vi "串口INI.vi"() -> ()   [LabVIEW 2019]
uses:
  <vilib>/Instr/_visa.llb/VISA Configure Serial Port (Instr).vi
panel:
  in  "启用终止符？":bool caption="启用终止符 (F)"
  in  "终止符":u8=10 format="%.0x"
  in  "超时":u32=10000 caption="超时（10秒）"
  in  "流控制":u16(ring) items=["无", "XON/XOFF", "RTS/CTS", "XON/XOFF & RTS/CTS", "DTR/DSR", "XON/XOFF & DTR/DSR"]
  in  "停止位":u16(ring)=10 items=["1.0"=10, "1.5"=15, "2.0"=20]
  in  "奇偶校验":enum16{"None", "Odd", "Even", "Mark", "Space"}(ring)
  in  "数据位":u16=8 min=5 max=8 step=1
  in  "波特率":u32=9600
  in  "VISA串口名称":refnum<visa-resource-name> caption="VISA资源名称"
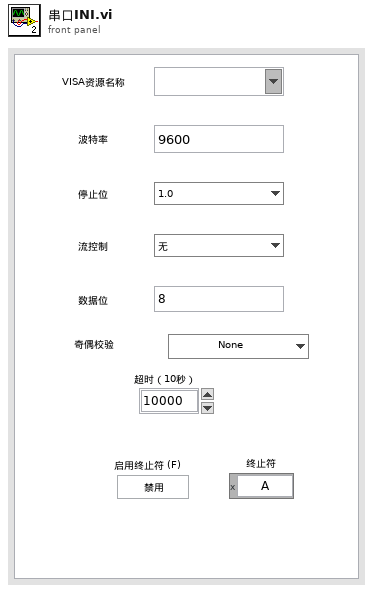
[diagram p1: front panel]
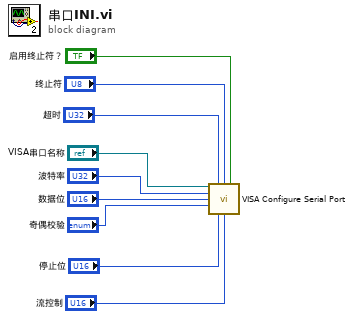
[diagram p0: block diagram]
diagram:
  n1 = call-poly "VISA Configure Serial Port"("VISA resource name"="VISA串口名称", "timeout (10sec)"="超时", "termination char\n(0xA = '\\n' = LF)"="终止符", "Enable Termination\nChar (T)"="启用终止符？", "baud rate (9600)"="波特率", "data bits (8)"="数据位", "parity (0:none)"="奇偶校验", "stop bits (10: 1 bit)"="停止位", "flow control (0:none)"="流控制") -> ()  [unwired: 5 in, 2 out]
